vi "SHGetFolderPath.vi"(4 "error in (no error)":errorcluster, 7 "Shell Folder (DESKTOP)":T1 items=["CSIDL_DESKTOP"=0, "CSIDL_PERSONAL"=5, "CSIDL_STARTUP"=7, "CSIDL_BITBUCKET"=10, "CSIDL_DRIVES"=17, "CSIDL_NETWORK"=18, "CSIDL_COMMON_PROGRAMS"=23, "CSIDL_COMMON_STARTUP"=24, "CSIDL_COMMON_DESKTOPDIRECTORY"=25, "CSIDL_PROGRAM_FILES"=38]) -> (0 "error out":errorcluster, 3 "FolderPath":path)   [LabVIEW 2011]
doc: "Gets the path to the Windows directory."
uses:
  SHFolderPaths.ctl
  SHELL32.DLL
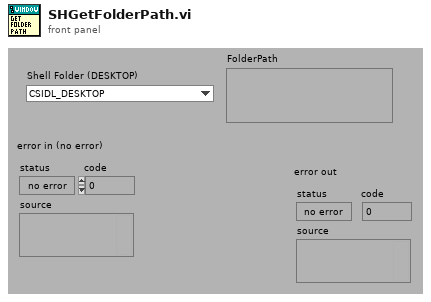
[diagram p1: front panel]
types:
  T1 = typedef "SHFolderPaths.ctl" = i32
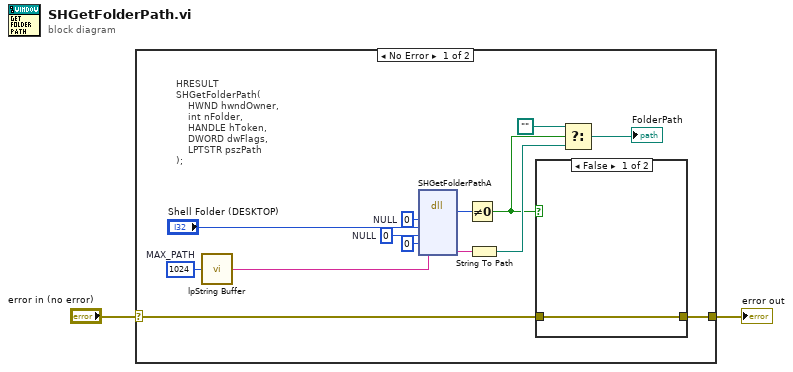
[diagram p0: block diagram]
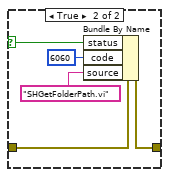
[diagram p2: hidden frame]
diagram:
  n1 = case shown="No Error" "error in (no error)" {
    selector: "error in (no error)" -> [w14 w23]
    tunnel: [w13 w23] -> w1
    frame No Error {
      w7 = 0  # NULL
      w8 = 0  # NULL
      w9 = 1024  # MAX_PATH
      # "HRESULT SHGetFolderPath(\n    HWND hwndOwner,\n    int nFolder,\n    HANDLE hToken,\n    DWORD dwFlags,\n    LPTSTR pszPath\n);"
      n2 = call "lpString Buffer.vi"("buffer size"=w9) -> ("string buffer"=w6:string)  [unwired: 4 out]
      n3 = dll-call lib="SHELL32.DLL" fn="SHGetFolderPathA"("hwndOwner"=w8, "nFolder"="Shell Folder (DESKTOP)", "hToken"=w7, "dwFlags"=u32 0, "pszPath"=w6) -> (w16:i32, "pszPath"=w4:string)  [unwired: 7 in, 2 out]
      n4 = Not Equal To 0?(x=w16) -> (x != 0?=w12:bool)
      n5 = String To Path(string=w4) -> (path=w15:path)
      n6 = case shown="False" w12 {
        selector: w12 -> [_ w18]
        tunnel: w14 -> [w17 w21]
        tunnel: [w17 w20] -> w13
        frame False {
        }
        frame True {
          n7 = Bundle By Name(cluster=w21, "status"=w18, "code"=6060, "source"="SHGetFolderPath.vi") -> (w20:errorcluster)
        }
      }
      n8 = Select(t=path "", s=w12, f=w15) -> (s? t:f=→"FolderPath":path)
    }
    frame Error {
    }
  }
  "error out" <- w1
